vi "led_test.vi"() -> ()   [LabVIEW 2019]
uses:
  <vilib>/rvi/Emulation/niFpgaGetClockAttributes.vi
  <vilib>/rvi/Emulation/niFpgaSctlEmulationGetInTimedLoop.vi
  <vilib>/rvi/Emulation/niFpgaEmulationReportErrorSimple.vi
  <vilib>/rvi/interface/RandomDataEmulation/niFpgaRandomDataHandleErrors.vi
  <vilib>/rvi/eio/common/nirviEmuTemplateMethod_errors.vi
  <vilib>/rvi/Emulation/niFpgaCriticalErrorInLSC.vi
  <vilib>/rvi/DataTransferAndStorage/Container/XNode/niFpgaContainer.xnode
  <vilib>/rvi/interface/RandomDataEmulation/nirviRandomDataFpgaReadWriteTemplate.vi
  <vilib>/eio/EIONode/EIONode.xnode
panel:
  in  "stop":bool
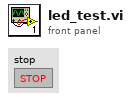
[diagram p1: front panel]
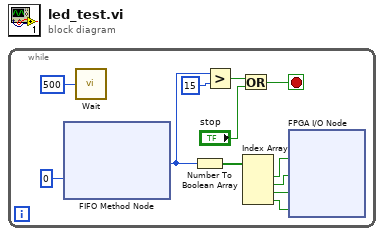
[diagram p0: block diagram]
diagram:
  n1 = while {
    stop <- w3 stop-if-true
    n2 = xnode ("FIFO Method Node")("Timeout"=0) -> ("Element"=w2:u8)  [unwired: 1 in, 2 out]
    n3 = call "Wait"("Count(mSec)"=u16 500) -> ()  [unwired: 1 out]
    n4 = Number To Boolean Array(number=w2) -> (Boolean array=w12:bool[])
    n5 = Greater?(x=w2, y=u8 15) -> (0:w5:bool)
    n6 = Or(x=w5, y="stop") -> (x .or. y?=w3:bool)
    n7 = Index Array(array=w12) -> (element #1=w11:bool, element #2=w10:bool, element #3=w9:bool, element #4=w8:bool)  [unwired: 4 in]
    n8 = xnode "FPGA I/O Node"("LED0"=w11, "LED1"=w10, "LED2"=w9, "LED3"=w8) -> ()  [unwired: 4 in, 4 out]
  }
